vi "niRFUtil WFM Complex Accumulator.vi"(7 "Waveform In":T1 {"y" format="%.2f"; "dx" format="%^.2e"; "x0" format="%^.2e"}) -> (8 "Waveform Out":T1 {"y" format="%.2f"; "dx" format="%^.2e"; "x0" format="%^.2e"})   [LabVIEW 2015, in "niRFUtil.lvlib"]
doc: "(c) Copyright 2006, National Instruments, Inc. This VI may not be duplicated, sold, or distributed without written consent from National Instruments."
uses:
  niRFUtil.lvlib
  Includes/niRFUtil INC Complex Waveform.ctl
  Includes/niRFUtil INC Complex Array.ctl
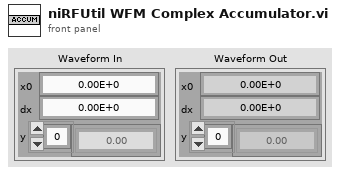
[diagram p1: front panel]
types:
  T1 = typedef "niRFUtil.lvlib/niRFUtil INC Complex Waveform.ctl" = cluster{"x0":dbl, "dx":dbl, "y":T2}
  T2 = typedef "niRFUtil.lvlib/niRFUtil INC Complex Array.ctl" = csg[]
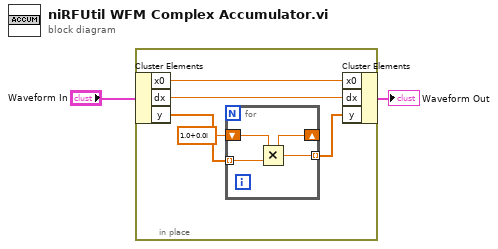
[diagram p0: block diagram]
diagram:
  n1 = in-place {
    n2 = in-place-cluster #1("Waveform In") -> ("x0"=w3:dbl, "dx"=w5:dbl, "y"=w6:T2)
    n3 = for {
      shift-right: [w8] -> _
      shift-left: csg 1.0+0.0i -> [w9]
      tunnel: w6 -> [w10] mode=indexing
      tunnel: [w8] -> w4 mode=indexing
      n4 = Multiply(x=w9, y=w10) -> (x*y=w8:csg)
    }
    n5 = in-place-cluster #1("x0"=w3, "dx"=w5, "y"=w4) -> (→"Waveform Out":T1)
  }
